vi "Handle Command.vi"(8 "error in":errorcluster, 10 "CMD in":refnum<class "Change Filter State CMD.lvclass">, 11 "Object In":refnum<class>) -> (0 "error out":errorcluster, 1 "Command Successful?":bool, 2 "CMD out":refnum<class "Change Filter State CMD.lvclass">, 3 "Object Out":refnum<class>)   [LabVIEW 2016, in "CRDS Lib.lvlib" / "Change Filter State CMD.lvclass"]
doc: "This VI will contain the code used to actually execute the request. If the request is successful, this will be indicated by the boolean output <b>Command Successful?</b>. The boolean output can then be used by the <b>Command Reply</b> which sends a reply if the reply queue is valid."
uses:
  Change Filter State CMD.lvclass
  Main/CRDS.lvclass
  Change Filter State CMD.lvclass/Change Filter State CMD.ctl
  Cell/CRDS Cell.lvclass/CRDS Cell.ctl
  Cell/Write filter.vi
  Main/Read Cells.vi
  Main/Write Cells.vi
  Cell/CRDS Cell.lvclass
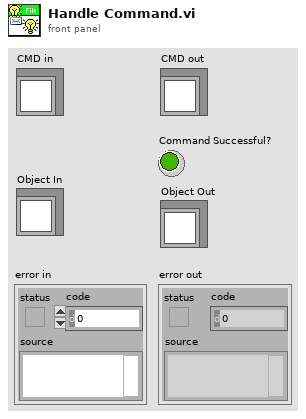
[diagram p1: front panel]
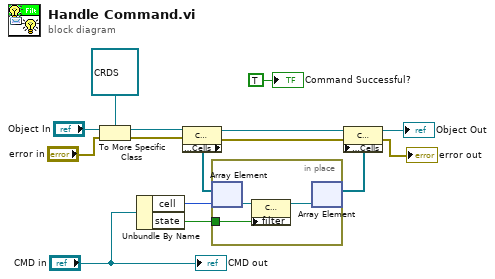
[diagram p0: block diagram]
diagram:
  n1 = To More Specific Class(target class=refnum<class "CRDS.lvclass"> refnum ("CRDS Lib.lvlib:CRDS"), reference="Object In", error in="error in") -> (specific class reference=w13:refnum<class "CRDS.lvclass">, error out=w12:errorcluster)
  n2 = Unbundle By Name("CMD in") -> ("cell"=w9:u8, "state"=w8:bool)
  n3 = property class="CRDS"(reference=w13, error in=w12) -> (reference out=w7:refnum<class "CRDS.lvclass">, error out=w2:errorcluster, "Data Access:Cells"=w11:refnum<class "CRDS Cell.lvclass">[])
  n4 = in-place {
    in-place-border: w8 -> [w17]
    n5 = in-place-array #1(w11, w9) -> (w18:refnum<class "CRDS Cell.lvclass">)
    n6 = property class="CRDS Cell"(reference=w18, "filter"=w17) -> (reference out=w16:refnum<class "CRDS Cell.lvclass">)  [unwired: 1 in, 1 out]
    n7 = in-place-array #1(w16) -> (w6:refnum<class "CRDS Cell.lvclass">[])  [unwired: 1 out]
  }
  n8 = property class="CRDS"(reference=w7, error in=w2, "Data Access:Cells"=w6) -> (reference out=→"Object Out":refnum<class "CRDS.lvclass">, error out=→"error out":errorcluster)
  "CMD out" <- "CMD in"
  "Command Successful?" <- TRUE ("Command Successful?")
